vi "Close.vi"(8 "error in (no error)":errorcluster, 11 "Tektronix PA1000 in":refnum<class "Tektronix PA1000.lvclass">) -> (0 "error out":errorcluster, 3 "Tektronix PA1000 out":refnum<class "Tektronix PA1000.lvclass">)   [LabVIEW 2014, in "Generic Power Analyzer.lvlib" / "Tektronix PA1000.lvlib" / "Tektronix PA1000.lvclass"]
uses:
  Tektronix PA1000.lvclass
  <instrlib>/Tektronix PA1000/Tektronix PA1000.lvlib
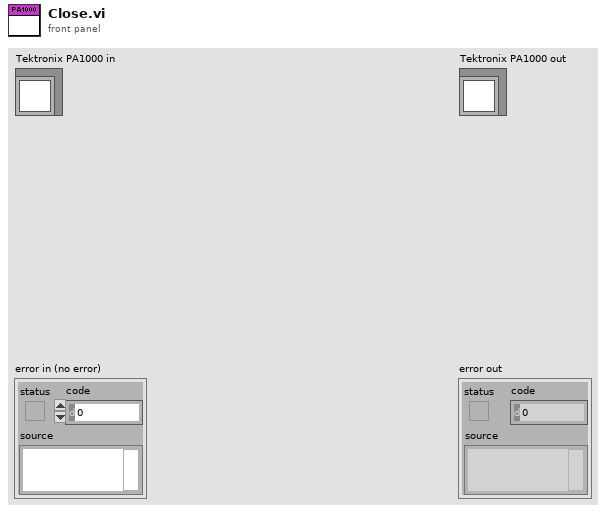
[diagram p1: front panel]
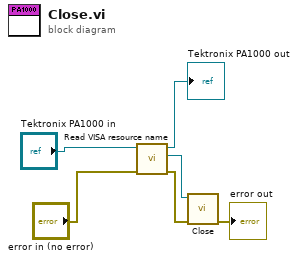
[diagram p0: block diagram]
diagram:
  n1 = call-dynamic "Read VISA resource name.vi"("error in (no error)"="error in (no error)", "Generic Instrument in"="Tektronix PA1000 in") -> ("error out"=w2:errorcluster, "VISA resource name"=w1:refnum<visa-resource-name>, "Generic Instrument out"=→"Tektronix PA1000 out":refnum<class "Tektronix PA1000.lvclass">)  [unwired: 7 in]
  n2 = call <instrlib>:"Close.vi"("error in (no error)"=w2, "VISA resource name"=w1) -> ("error out"=→"error out":errorcluster)  [unwired: 9 in]
